vi "NanotecSMCPD.move axis absolute.vi"(0 "i ref in":refnum<vi>, 1 "axis":i32, 2 "absPosition [unit]":dbl, 3 "ms timeout (10000)":i32=10000, 5 "error in (no error)":errorcluster) -> (14 "i ref out":refnum<vi>, 17 "timed out":bool, 19 "error out":errorcluster)   [LabVIEW 2014, in "NanotecSMCPD.lvlib"]
doc: "Moves the specified axis to the absolute position specified."
uses:
  NanotecSMCPD.lvlib
  CSCore/CSSystem/CoreDefs/CoreDefs.error_type.ctl
  CSCore/CSSystem/CoreDefs/CoreDefs.error_severity.ctl
  CSCore/CSApplicationBaseClasses/MotorBase/MotorBase.directionType.ctl
  CSCore/CSApplicationBaseClasses/MotorBase/MotorBase.serviceType.ctl
  CSCore/CSApplicationBaseClasses/MotorBase/MotorBase.statusType.ctl
  CSlibraries/UtilityLib/UtilityLib.valueStatus.ctl
  CSCore/CSApplicationBaseClasses/DeviceBase/DeviceBase.lvlib
  CSCore/CSSystem/CoreLib/CoreLib.lvlib
  CSCore/CSApplicationBaseClasses/MotorBase/MotorBase.lvlib
  CSlibraries/UtilityLib/UtilityLib.lvlib
  CSinstr.lib/NanotecSMCPD/NanotecSMCPDDriver.lvlib
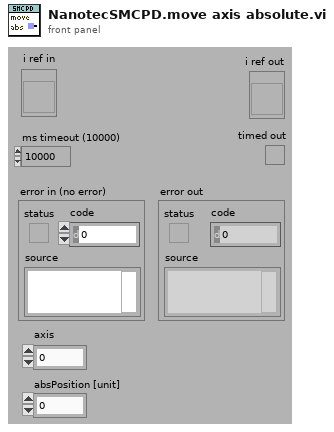
[diagram p1: front panel]
types:
  T1 = typedef "CoreDefs.error_severity.ctl" = enum16{"undefined", "information", "warning", "error", "fatal"}
  T2 = typedef "CoreDefs.error_type.ctl" = enum16{"no error", "can't load process", "can't unload process", "process does not exist", "can't install process", "can't remove process", "unknown function", "time out", "can't execute function", "duplicate queue name", "super not found", "caller queue invalid", "can't ping process", "unknown error", "VISA Error", "VISA timeout", "GPIB timeout", "GPIB error", "communication error", "data type mismatch", "can't read data from OPC server", "can't write data to OPC server", "OET error", "function not implemented", "process already exists", "invalid Shared Variable name", "error writing Shared Variable", "error reading Shared Variable", "invalid client name", "corrupt database", "unknown class", "call not authorized", "parameter out of range", "OET timeout: can't get data to modify", "invalid queue name", "requested operation incompatible with current state", "event undefined", "event disabled", "state undefined", "caller is not a friend", "EventBuilder: bad eventID", "EventBuilder: no DAQ devices", "a thread must not stop itself", "UNUSED ELEMENT4", "DiscArchiver: eventData incomplete", "DiscArchiver: eventData does not belong to run", "DiscArchiver: can't open file", "DiscArchiver: can't write to file", "DiscArchiver: available disc space low", "can't acquire semaphore", "error reading data from database", "notifier object is not existing", "can't register process", "can't unregister process", "illegal event type", "object disabled", "object already exists", "can't change state", "Instrument not found", "no connection to remote node", "invalid reference", "N/A", "UNUSED ELEMENT 1", "element not found", "illegal TCP/IP connection detected", "object does not exist", "invalid access ID", "unknown CS system", "invalid privilige", "unsupported data type", "unsupported server type", "IO server already exists", "Shared Variable already exists"}
  T3 = typedef "UtilityLib.lvlib/UtilityLib.valueStatus.ctl" = enum16{"no info available", "stand by/off", "on", "warning", "alarm/malfunction", "not implemented", "user action required", "important information", "system default", "control default", "indicator default", "button default"}
  T4 = typedef "MotorBase.lvlib/MotorBase.serviceType.ctl" = enum16{"onOff", "startVelocity", "stopVelocity", "acceleration", "rangeMin", "rangeMax", "status", "position"}
  T5 = typedef "MotorBase.lvlib/MotorBase.directionType.ctl" = enum16{"unknown", "update actual value", "update nominal value", "update both"}
  T6 = typedef "MotorBase.lvlib/MotorBase.statusType.ctl" = u32
  T7 = typedef "NanotecSMCPD.lvlib/NanotecSMCPD.i attribute.ctl" = cluster{"referencing":bool[], "stop":bool[], "AutoHalt ID":i32, "MethodQueue":refnum<queue>, "Referenced1Time?":bool[], "LastCommand ID":i32}
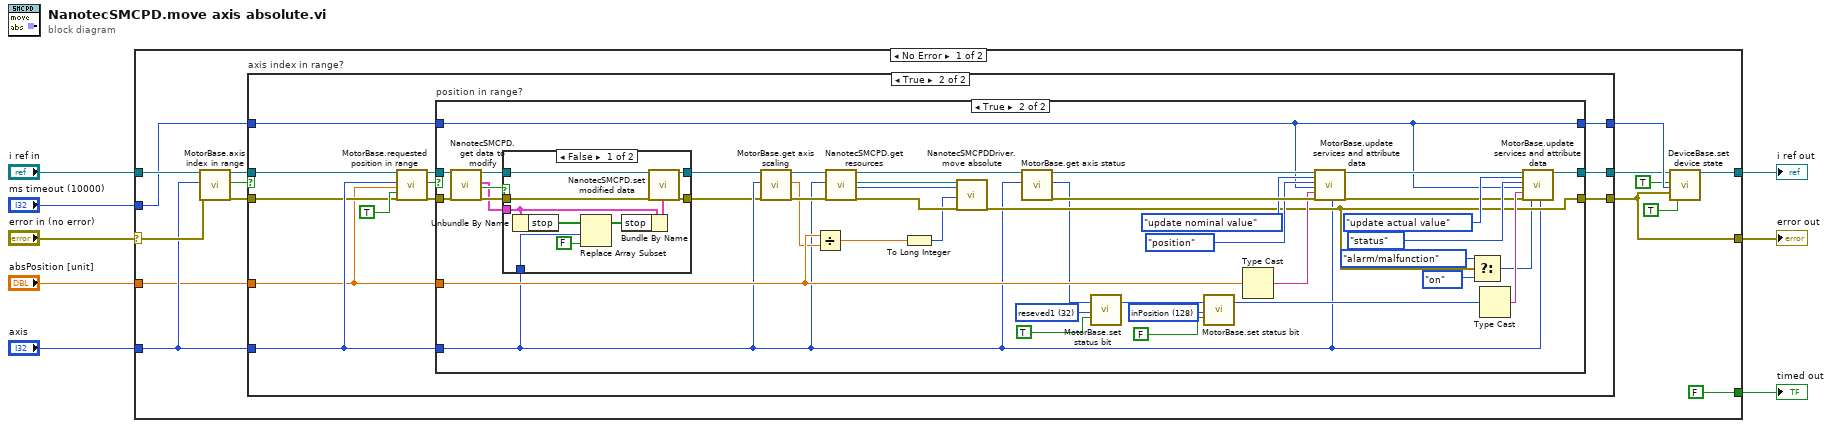
[diagram p0: block diagram]
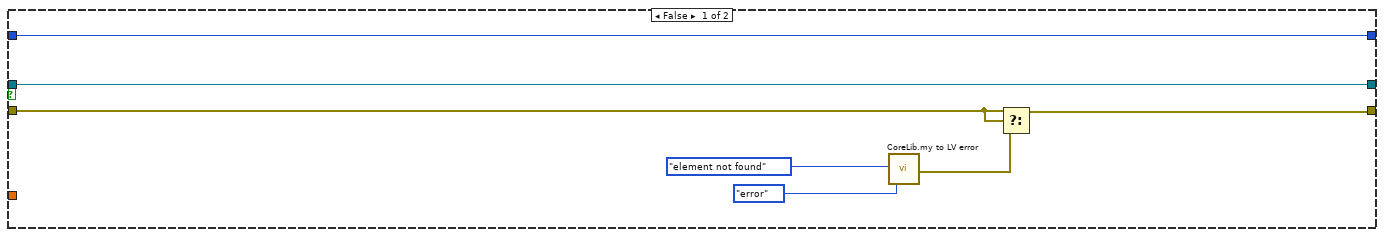
[diagram p2: hidden frame]
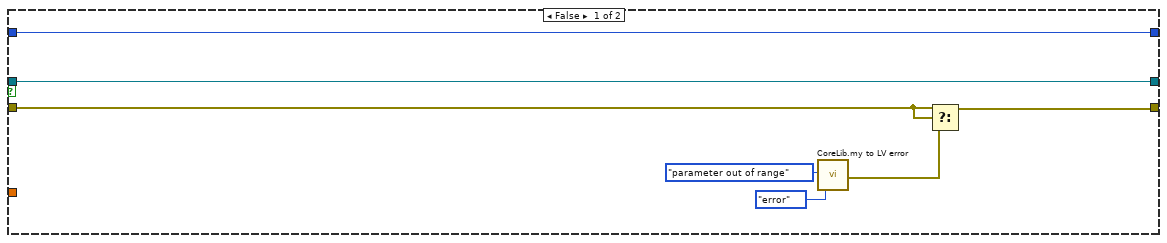
[diagram p3: hidden frame]
diagram:
  n1 = case shown="No Error" "error in (no error)" {
    selector: "error in (no error)" -> [w16 w104]
    tunnel: "ms timeout (10000)" -> [w13 _]
    tunnel: "i ref in" -> [w17 w105]
    tunnel: [w15 w104] -> w5
    tunnel: "axis" -> [w14 _]
    tunnel: [w12 w105] -> w3
    tunnel: "absPosition [unit]" -> [w11 _]
    tunnel: [FALSE _] -> w1
    frame No Error {
      n2 = call "MotorBase.axis index in range.vi"("i ref in"=w17, "axisIndex"=w14, "error in (no error)"=w16) -> ("i ref out"=w21:refnum<vi>, "in range"=w20:bool, "error out"=w22:errorcluster)  [unwired: 14 in]
      n3 = case "axis index in range?" shown="True" w20 {
        tunnel: [w30 w42] -> w19
        tunnel: [w27 w41] -> w15
        tunnel: w13 -> [w24 w40]
        tunnel: w14 -> [_ w34]
        tunnel: w21 -> [w30 w33]
        tunnel: w22 -> [w28 w32]
        tunnel: [w24 w35] -> w23
        tunnel: w11 -> [_ w31]
        frame False {
          n4 = call "CoreLib.my to LV error.vi"("ErrorTypes"=CoreDefs.error_type."element not found", "severityLevel"=CoreDefs.error_severity."error") -> ("myErrorCluster"=w26:errorcluster)  [unwired: 16 in, 1 out]
          n5 = Select(t=w28, s=w28, f=w26) -> (s? t:f=w27:errorcluster)
        }
        frame True {
          n6 = call "MotorBase.requested position in range.vi"("i ref in"=w33, "axisIndex"=w34, "reqPosition"=w31, "absolute"=TRUE, "error in (no error)"=w32) -> ("i ref out"=w38:refnum<vi>, "in range"=w36:bool, "error out"=w37:errorcluster)  [unwired: 12 in]
          n7 = case "position in range?" shown="True" w36 {
            tunnel: [w49 w90] -> w42
            tunnel: [w44 w69] -> w41
            tunnel: w40 -> [w43 w80]
            tunnel: w34 -> [_ w53]
            tunnel: w31 -> [_ w71]
            tunnel: w38 -> [w49 w59]
            tunnel: w37 -> [w45 w58]
            tunnel: [w43 w80] -> w35
            frame False {
              n8 = call "CoreLib.my to LV error.vi"("ErrorTypes"=CoreDefs.error_type."parameter out of range", "severityLevel"=CoreDefs.error_severity."error") -> ("myErrorCluster"=w47:errorcluster)  [unwired: 16 in, 1 out]
              n9 = Select(t=w45, s=w45, f=w47) -> (s? t:f=w44:errorcluster)
            }
            frame True {
              w62 = T6 32 items=["motorEnabled"=1, "negativeLimitSwitchActive"=2, "positiveLimitSwitchActive"=4, "limitSwitchesEnabled"=8, "limitSwitchesAreNormallyClosed"=16, "reseved1"=32, "referenced"=64, "inPosition"=128, "reserved2"=256, "reserved3"=512, "reserved4"=1024, "reserved5"=2048, "error"=4096, "reserved6"=8192, "reserved7"=16384, "reserved8"=32768, "user defined1"=65536, "user defined2"=131072, "user defined3"=262144, "user defined4"=524288, "user defined5"=1048576, "user defined6"=2097152, "user defined7"=4194304, "user defined8"=8388608, "user defined9"=16777216, "user defined10"=33554432, "user defined11"=67108864, "user defined12"=134217728, "user defined13"=268435456, "user defined14"=536870912, "user defined15"=1073741824, "user defined16"=2147483648] ("statusBit")
              w75 = T6 128 items=["motorEnabled"=1, "negativeLimitSwitchActive"=2, "positiveLimitSwitchActive"=4, "limitSwitchesEnabled"=8, "limitSwitchesAreNormallyClosed"=16, "reseved1"=32, "referenced"=64, "inPosition"=128, "reserved2"=256, "reserved3"=512, "reserved4"=1024, "reserved5"=2048, "error"=4096, "reserved6"=8192, "reserved7"=16384, "reserved8"=32768, "user defined1"=65536, "user defined2"=131072, "user defined3"=262144, "user defined4"=524288, "user defined5"=1048576, "user defined6"=2097152, "user defined7"=4194304, "user defined8"=8388608, "user defined9"=16777216, "user defined10"=33554432, "user defined11"=67108864, "user defined12"=134217728, "user defined13"=268435456, "user defined14"=536870912, "user defined15"=1073741824, "user defined16"=2147483648] ("service")
              n10 = call "NanotecSMCPD.get data to modify.vi"("i ref in"=w59, "error in (no error)"=w58) -> ("i ref out"=w56:refnum<vi>, "i attribute"=w54:T7, "timed out"=w57:bool, "error out"=w55:errorcluster)  [unwired: 14 in]
              n11 = case shown="False" w57 {
                tunnel: w56 -> [w101 w103]
                tunnel: [w100 w103] -> w52
                tunnel: w55 -> [w99 w102]
                tunnel: [w98 w102] -> w51
                tunnel: w54 -> [w97 _]
                tunnel: w53 -> [w93 _]
                frame False {
                  n12 = Unbundle By Name(w97) -> ("stop"=w95:bool[])
                  n13 = Replace Array Subset(array=w95, new element=FALSE ("new element/subarray"), index=w93) -> (w94:bool[])
                  n14 = Bundle By Name(cluster=w97, "stop"=w94) -> (w96:T7)
                  n15 = call "NanotecSMCPD.set modified data.vi"("i ref in"=w101, "i attribute"=w96, "error in (no error)"=w99) -> ("i ref out"=w100:refnum<vi>, "error out"=w98:errorcluster)  [unwired: 15 in]
                }
                frame True {
                }
              }
              n16 = call "MotorBase.get axis scaling.vi"("i ref in"=w52, "axisIndex"=w53, "error in (no error)"=w51) -> ("i ref out"=w73:refnum<vi>, "scaling"=w70:dbl, "error out"=w72:errorcluster)  [unwired: 14 in]
              n17 = Divide(x=w71, y=w70) -> (x/y=w50:dbl)
              n18 = call "NanotecSMCPD.get resources.vi"("i ref in"=w73, "axisNumber"=w53, "error in (no error)"=w72) -> ("i ref out"=w77:refnum<vi>, "VISA resource"=w79:refnum<visa-resource-name>, "address"=w65:i32, "error out"=w78:errorcluster)  [unwired: 13 in]
              n19 = To Long Integer(number=w50) -> (32bit integer=w64:i32)
              n20 = call "NanotecSMCPDDriver.move absolute.vi"("VISA resource name"=w79, "contollerID"=w65, "nOfSteps [uSteps]"=w64, "error in (no error)"=w78) -> ("error out"=w69:errorcluster)  [unwired: 13 in, 2 out]
              n21 = call "MotorBase.get axis status.vi"("i ref in"=w77, "axisIndex"=w53) -> ("i ref out"=w87:refnum<vi>, "status"=w63:T6, "error out"=w84:errorcluster)  [unwired: 15 in]
              n22 = call "MotorBase.set status bit.vi"("status"=w63, "statusBit"=w62, "setBit"=TRUE) -> ("status out"=w61:T6)  [unwired: 16 in]
              n23 = call "MotorBase.set status bit.vi"("status"=w61, "statusBit"=w75, "setBit"=FALSE) -> ("status out"=w76:T6)  [unwired: 16 in]
              n24 = Type Cast(x=w71) -> (*(type *) &x=w83:string)  [unwired: 1 in]
              n25 = call "MotorBase.update services and attribute data.vi"("i ref in"=w87, "direction"=MotorBase.directionType."update nominal value", "service"=MotorBase.serviceType."position", "ms timeout (10000)"=w80, "value"=w83, "error in (no error)"=w84, "axisNumber"=w53) -> ("i ref out"=w86:refnum<vi>, "error out"=w85:errorcluster)  [unwired: 10 in, 1 out]
              n26 = Select(t=UtilityLib.valueStatus."alarm/malfunction", s=w69, f=UtilityLib.valueStatus."on" ("quality")) -> (s? t:f=w66:T3)
              n27 = Type Cast(x=w76) -> (*(type *) &x=w91:string)  [unwired: 1 in]
              n28 = call "MotorBase.update services and attribute data.vi"("i ref in"=w86, "direction"=MotorBase.directionType."update actual value", "service"=MotorBase.serviceType."status", "ms timeout (10000)"=w80, "value"=w91, "error in (no error)"=w85, "quality"=w66, "axisNumber"=w53) -> ("i ref out"=w90:refnum<vi>)  [unwired: 9 in, 2 out]
            }
          }
        }
      }
      n29 = call "DeviceBase.set device state.vi"("i ref in"=w19, "implicit"=TRUE, "ms timeout (10000)"=w23, "device error"=w15, "mayResetError (FALSE)"=TRUE) -> ("i ref out"=w12:refnum<vi>)  [unwired: 12 in, 2 out]
    }
    frame Error {
    }
  }
  "error out" <- w5
  "i ref out" <- w3
  "timed out" <- w1
